vi "Apply Speed Limit.vi"(8 "error in":errorcluster, 10 "Speed In":dbl, 11 "Gantry in":refnum<class "Gantry Class.lvclass">) -> (0 "error out":errorcluster, 2 "Speed Limited":dbl, 3 "Gantry out":refnum<class "Gantry Class.lvclass">)   [LabVIEW 2011, in "Gantry Class.lvclass"]
uses:
  Gantry Class.lvclass
  Gantry Class.lvclass/Gantry Class.ctl
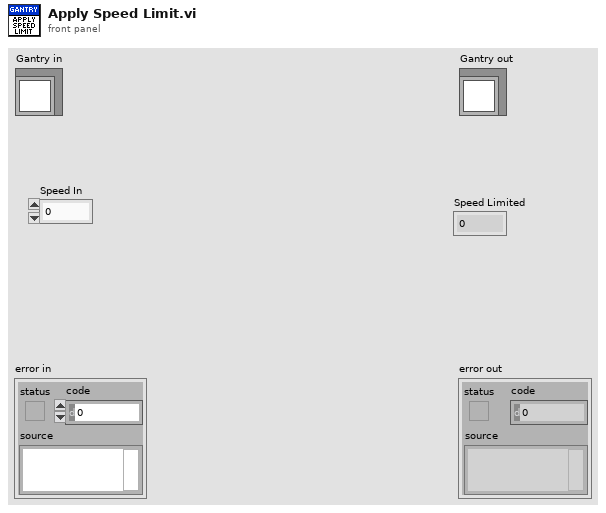
[diagram p1: front panel]
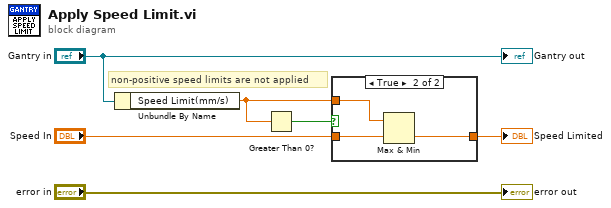
[diagram p0: block diagram]
diagram:
  # "non-positive speed limits are not applied"
  n1 = Unbundle By Name("Gantry in") -> ("Speed Limit(mm/s)"=w2:dbl)
  n2 = Greater Than 0?(x=w2) -> (x > 0?=w3:bool)
  n3 = case shown="True" w3 {
    tunnel: "Speed In" -> [w7 w9]
    tunnel: w2 -> [_ w10]
    tunnel: [w7 w8] -> w1
    frame False {
    }
    frame True {
      n4 = Max & Min(x=w10, y=w9) -> (min(x,y)=w8:dbl)  [unwired: 1 out]
    }
  }
  "Speed Limited" <- w1
  "error out" <- "error in"
  "Gantry out" <- "Gantry in"
